vi "sequence_practice.vi"() -> ()   [LabVIEW 2018]
panel:
  out "웨이브폼 차트 2":dbl(graph)
  in  "정지":bool
  out "웨이브폼 차트":dbl[](graph)
  in  "불리언":bool
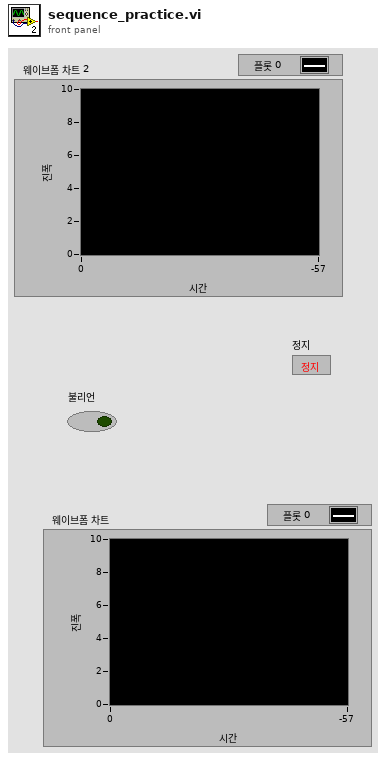
[diagram p1: front panel]
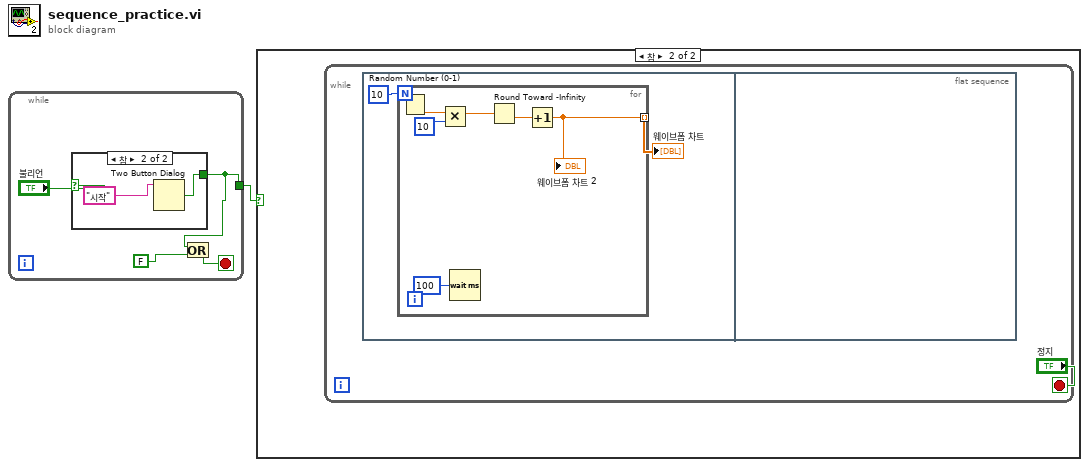
[diagram p0: block diagram]
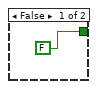
[diagram p3: hidden frame]
diagram:
  n1 = while {
    tunnel: [w2] -> w1
    stop <- w3 stop-if-true
    n2 = case shown="참" "불리언" {
      tunnel: [FALSE w8] -> w2
      frame False {
      }
      frame True {
        n3 = Two Button Dialog(message="시작") -> (T button?=w8:bool)  [unwired: 2 in]
      }
    }
    n4 = Or(x=w2, y=FALSE) -> (x .or. y?=w3:bool)
  }
  n5 = case shown="참" w1 {
    frame False {
    }
    frame True {
      n6 = while {
        stop <- "정지" stop-if-true
        n7 = flat-sequence {
          frame #0 {
            n8 = for {
              N: 10 -> [_]
              tunnel: [w12] -> w10 mode=indexing
              n9 = Random Number (0-1)() -> (number: 0 to 1=w16:dbl)
              n10 = Multiply(x=w16, y=10) -> (x*y=w15:dbl)
              n11 = Wait (ms)(milliseconds to wait=u32 100 ("대기 시간 (ms)")) -> ()  [unwired: 1 out]
              n12 = Round Toward -Infinity(1:w15) -> (0:w14:dbl)
              n13 = Increment(x=w14) -> (x+1=w12:dbl)
              "웨이브폼 차트 2" <- w12
            }
            "웨이브폼 차트" <- w10
          }
          frame #1 {
          }
        }
      }
    }
  }
